vi "_Look Up SharedString.vi"(8 "error in":errorcluster, 9 "Index":string, 10 "WorkbookPart":refnum<k24>) -> (0 "error out":errorcluster, 2 "String Value":string)   [LabVIEW 2021, in "Open Xml.lvlib"]
uses:
  Open Xml.lvlib
  D:/git/Open-Xml-LabVIEW/DocumentFormat.OpenXml.dll
  DocumentFormat.OpenXml.dll
  D:/git/Open-Xml-LabVIEW/DocumentFormat.OpenXml.Framework.dll
  DocumentFormat.OpenXml.Framework.dll
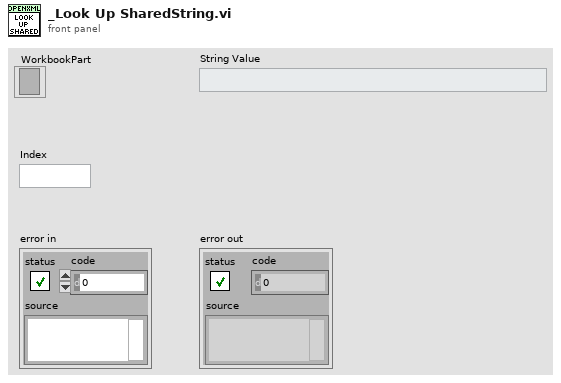
[diagram p1: front panel]
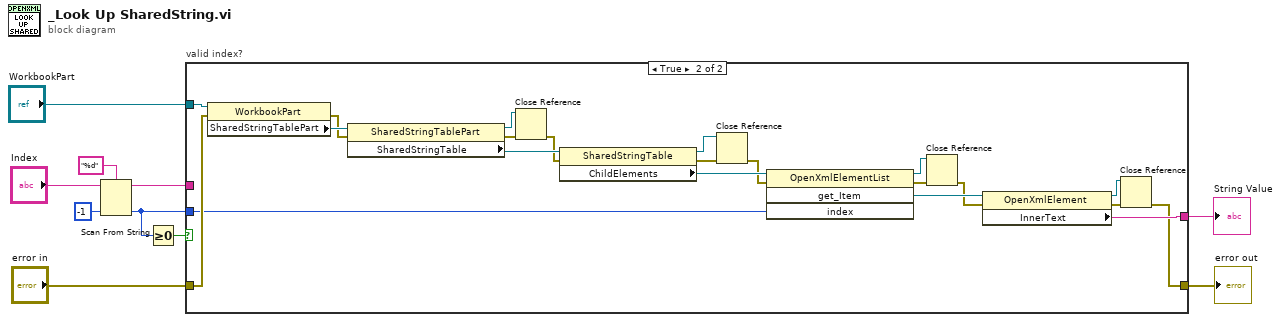
[diagram p0: block diagram]
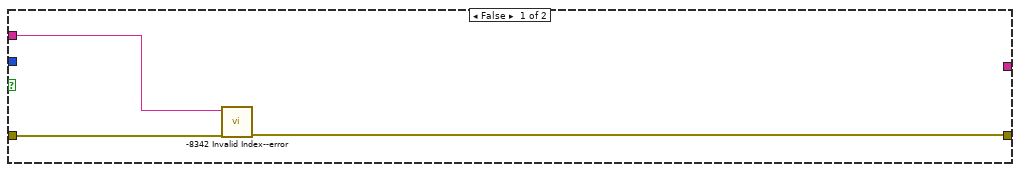
[diagram p2: hidden frame]
diagram:
  n1 = Scan From String(format string="%d", input string="Index", default 1=-1) -> (remaining string=w4:string, output 1=w6:i32)  [unwired: 2 in, 2 out]
  n2 = Greater Or Equal To 0?(x=w6) -> (x >= 0?=w7:bool)
  n3 = case "valid index?" shown="True" w7 {
    tunnel: w6 -> [_ w28]
    tunnel: [w13 w24] -> w5
    tunnel: w4 -> [w12 _]
    tunnel: "WorkbookPart" -> [_ w32]
    tunnel: "error in" -> [w11 w31]
    tunnel: [_ w26] -> w1
    frame False {
      n4 = call "-8342 Invalid Index--error.vi"("error in"=w11, "Index"=w12) -> ("error out"=w13:errorcluster)  [unwired: 9 in]
    }
    frame True {
      n5 = property class="WorkbookPart"(reference=w32, error in=w31) -> (error out=w16:errorcluster, "SharedStringTablePart"=w34:refnum<k24>)  [unwired: 1 out]
      n6 = property class="SharedStringTablePart"(reference=w34, error in=w16) -> (reference out=w17:refnum<k24>, error out=w30:errorcluster, "SharedStringTable"=w33:refnum<k24>)
      n7 = Close Reference(reference=w17, error in (no error)=w30) -> (error out=w18:errorcluster)
      n8 = property class="SharedStringTable"(reference=w33, error in=w18) -> (reference out=w19:refnum<k24>, error out=w21:errorcluster, "ChildElements"=w29:refnum<k24>)
      n9 = Close Reference(reference=w19, error in (no error)=w21) -> (error out=w20:errorcluster)
      n10 = invoke class="OpenXmlElementList" method="get_Item"(reference=w29, error in=w20, "index"=w28) -> (reference out=w14:refnum<k24>, error out=w27:errorcluster, "get_Item"=w23:refnum<k24>)  [unwired: 1 in, 1 out]
      n11 = Close Reference(reference=w14, error in (no error)=w27) -> (error out=w15:errorcluster)
      n12 = property class="OpenXmlElement"(reference=w23, error in=w15) -> (reference out=w22:refnum<k24>, error out=w25:errorcluster, "InnerText"=w26:string)
      n13 = Close Reference(reference=w22, error in (no error)=w25) -> (error out=w24:errorcluster)
    }
  }
  "error out" <- w5
  "String Value" <- w1
